vi "R_W_sqlDatabase.vi"(9 "Sentencia SQL":string, 10 "Get Data/Instert Data":T1(ring), 11 "Connect UDL":string="sql1") -> (2 "Data":string[][](array[string]))   [LabVIEW 2019]
panel:
  in  "Column":i32=1
  in  "Row":i32
  out "Elemento extraído":string
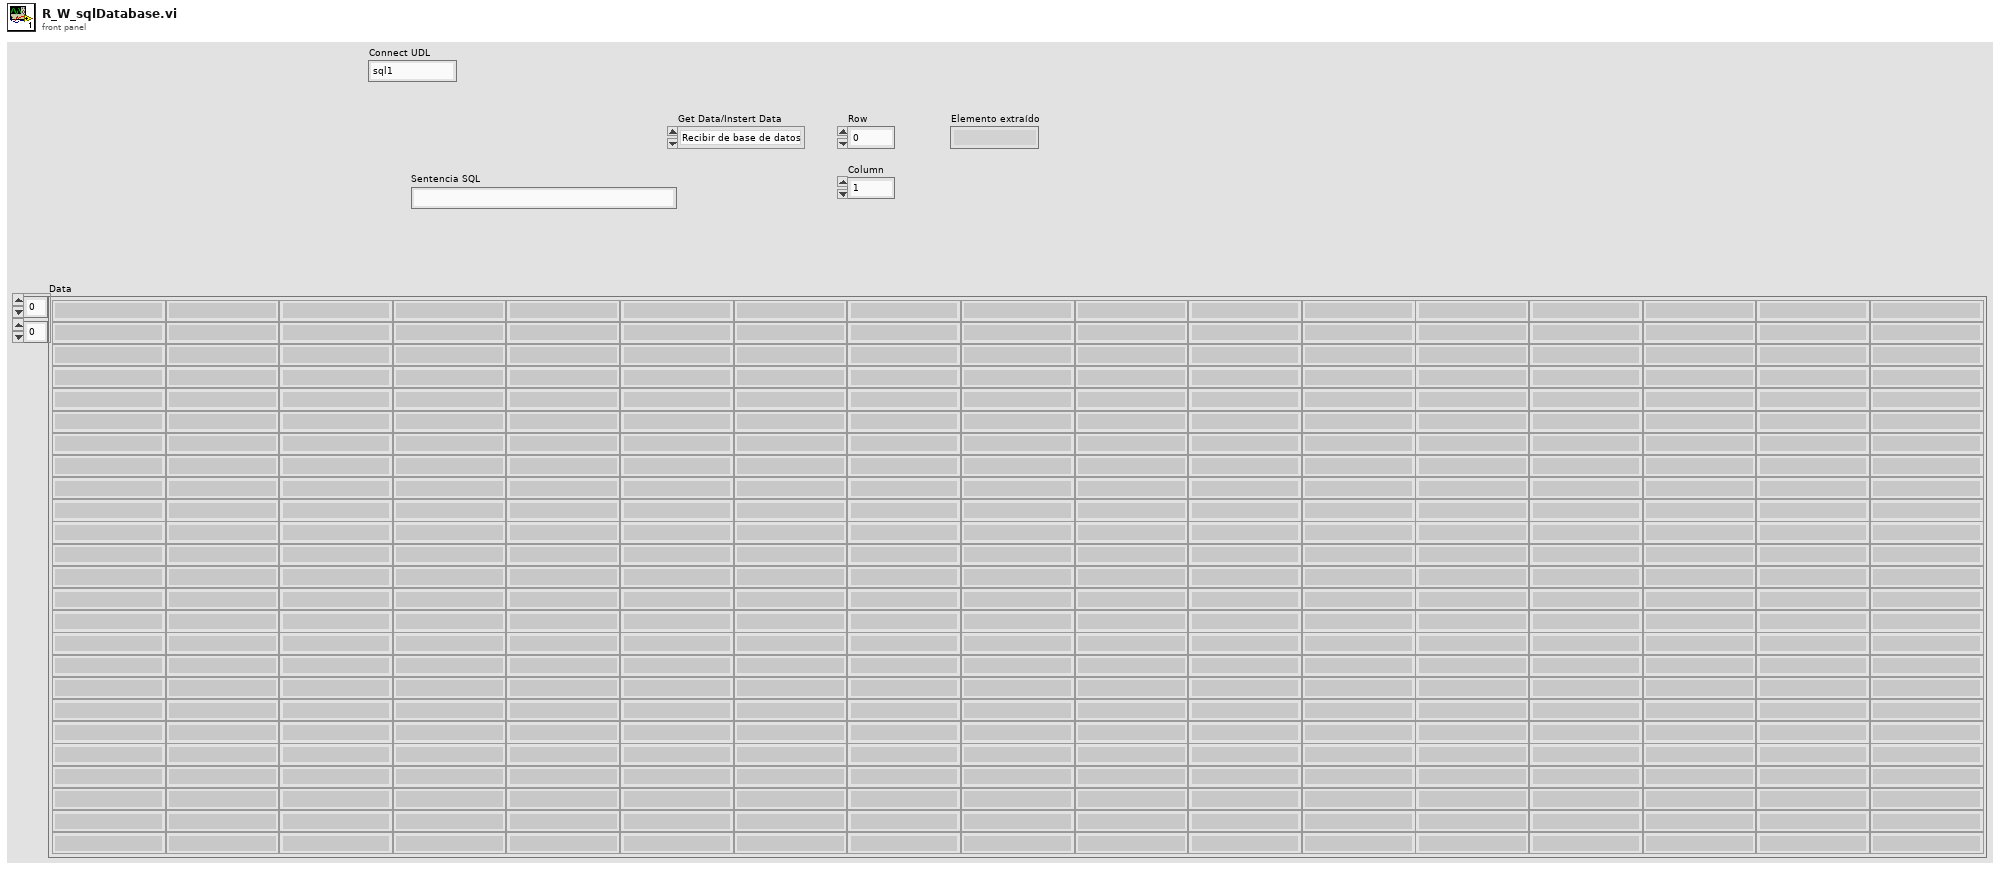
[diagram p1: front panel]
types:
  T1 = enum16{"Recibir de base de datos", "Escribir en base de datos"}
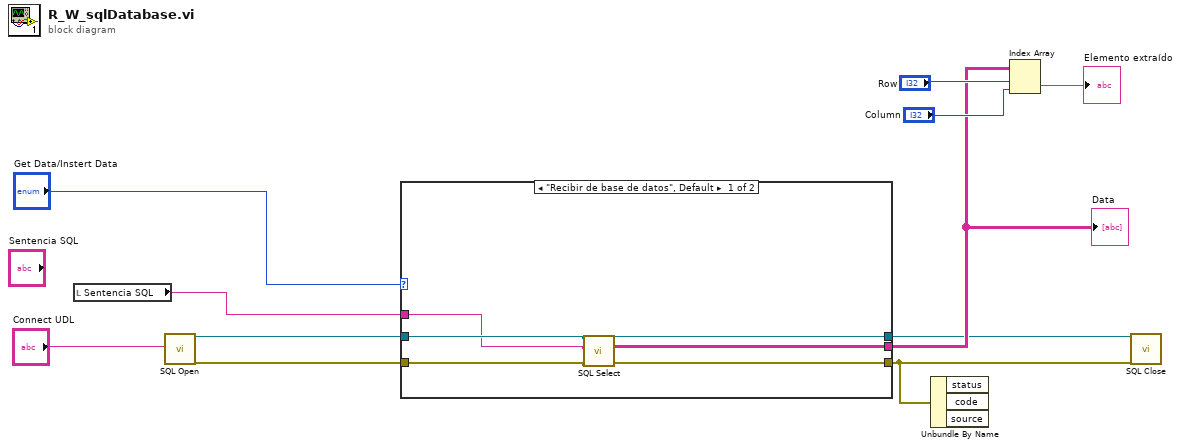
[diagram p0: block diagram]
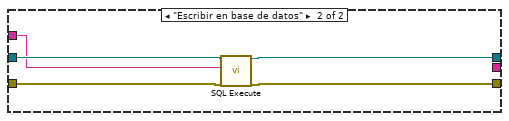
[diagram p2: hidden frame]
diagram:
  n1 = local read "Sentencia SQL"() -> (w6:string)
  n2 = call "SQL Open.vi"("ConnectionString In"="Connect UDL") -> ("Connection Out"=w4:refnum<k7>, "Error out"=w3:errorcluster)  [unwired: 17 in]
  n3 = case shown="\"Recibir de base de datos\", Default" "Get Data/Instert Data" {
    tunnel: w6 -> [w12 w18]
    tunnel: [w15 _] -> w8
    tunnel: w4 -> [w17 w19]
    tunnel: w3 -> [w13 w22]
    tunnel: [w16 w20] -> w2
    tunnel: [w14 w21] -> w1
    frame "Recibir de base de datos", Default {
      n4 = call "SQL Select.vi"("Connection In"=w17, "SQL Query"=w12, "Error in (no error)"=w13) -> ("Connection Out"=w16:refnum<k7>, "Data"=w15:string[][], "Error out"=w14:errorcluster)  [unwired: 14 in]
    }
    frame "Escribir en base de datos" {
      n5 = call "SQL Execute.vi"("Connection In"=w19, "SQL Query"=w18, "Error in (no error)"=w22) -> ("Connection Out"=w20:refnum<k7>, "Error out"=w21:errorcluster)  [unwired: 15 in]
    }
  }
  "Data" <- w8
  n6 = Unbundle By Name(w1) -> ()  [unwired: 3 out]
  n7 = Index Array(array=w8, index (row)="Row", index (col)="Column") -> (element=→"Elemento extraído":string)
  n8 = call "SQL Close.vi"("Connection In"=w2, "Error in (no error)"=w1) -> ()  [unwired: 17 in, 1 out]
